vi "simple approval test.vi"   [LabVIEW 2020]
uses:
  <vilib>/SAS/Approval Tests/Approval Tests/Options/Options.lvclass/Options.ctl
  <vilib>/SAS/Approval Tests/Approval Tests/Naming Data/Naming Data.lvclass/Naming Data.ctl
  dd95422e-ebbf-4799-9ae6-cf0dc6a18170.vi
  dd95422e-ebbf-4799-9ae6-cf0dc6a18170.vi/500b534b-d6f0-4fa5-90b2-c40158375321.vi
  <vilib>/SAS/Approval Tests/Approval Tests/Update Test Name if Not Defined.vi
  dd95422e-ebbf-4799-9ae6-cf0dc6a18170.vi/500b534b-d6f0-4fa5-90b2-c40158375321.vi/93c5622b-9fb7-41e0-8c76-3fde37e94e34.vi
  <vilib>/SAS/Approval Tests/Approval Tests/Verify Core.vi
  <vilib>/SAS/Approval Tests/Approval Tests/Options/Read Scrubber.vi
  <vilib>/SAS/Approval Tests/Approval Tests/Naming Data/Read Test VI Name.vi
  <vilib>/SAS/Approval Tests/Approval Tests/Naming Data/Write Test VI Name.vi
  dd95422e-ebbf-4799-9ae6-cf0dc6a18170.vi/500b534b-d6f0-4fa5-90b2-c40158375321.vi/93c5622b-9fb7-41e0-8c76-3fde37e94e34.vi/04cb982b-2eda-40d0-8d7e-90f8e0b569b2.vi
  <vilib>/SAS/Approval Tests/Approval Tests/Options/Read Namer.vi
  <vilib>/SAS/Approval Tests/Approval Tests/Options/Read Naming Data.vi
  <vilib>/SAS/Approval Tests/Approval Tests/Options/Read Reporter.vi
  <vilib>/SAS/Approval Tests/Approval Tests/conv EOL.vi
  <vilib>/Utility/libraryn.llb/Check if File or Folder Exists.vi
  <vilib>/SAS/Approval Tests/Approval Tests/Reporter/Report.vi
  <vilib>/addons/_JKI Toolkits/Caraya/classes/Assert/Assert.vi
  <vilib>/addons/_JKI Toolkits/Caraya/classes/Assert/Assert True.vi
  <vilib>/SAS/Approval Tests/Approval Tests/Options/Options.lvclass
  <vilib>/SAS/Approval Tests/Approval Tests/Scrubber/Scrubber.lvclass
  <vilib>/SAS/Approval Tests/Approval Tests/Namer/Namer.lvclass
  <vilib>/SAS/Approval Tests/Approval Tests/Naming Data/Naming Data.lvclass
  <vilib>/SAS/Approval Tests/Approval Tests/Reporter/Reporter.lvclass
  <vilib>/addons/_JKI Toolkits/Caraya/classes/Test/Test.lvclass
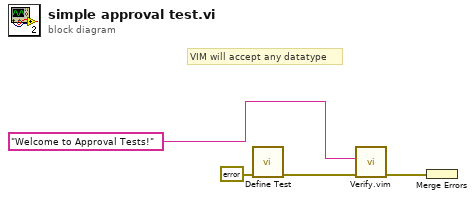
[diagram p0: block diagram]
diagram:
  # "VIM will accept any datatype"
  n1 = call <vilib>:"Define Test.vi"("error in (no error)"=errorcluster {"status"=FALSE, "code"=0, "source"=""}) -> ("error out"=w3:errorcluster)  [unwired: 9 in, 1 out]
  n2 = call "Verify.vim"("error in"=w3, "Test Data"="Welcome to Approval Tests!") -> ("error out"=w4:errorcluster)  [unwired: 8 in, 1 out]
  n3 = Merge Errors(w4) -> ()  [unwired: 1 out]
